vi "Shoot High Goal State Machine.vi"   [LabVIEW 2013]
uses:
  typedefs/fg_typedef.ctl
  typedefs/DevRef Type.ctl
  typedefs/subStates.ctl
  typedefs/singleUseSubstate.ctl
  <vilib>/Rock Robotics/WPI/Solenoid/WPI_SolenoidValue.ctl
  <vilib>/Rock Robotics/WPI/Solenoid/WPI_SolenoidGetEnum.vi
panel:
  # "A State Machine to Handle a High Goal Shot"
types:
  T1 = typedef "DevRef Type.ctl" = enum16{"Shooter Solenoid", "Latch Solenoid", "Right Up Sensor", "Right Down Sensor", "Hold Sensor", "2 Ball Switch", "Arm Encoder"}
  T2 = typedef "fg_typedef.ctl" = enum16{"Get", "Set"}
  T3 = typedef "subStates.ctl" = enum16{"null", "wait", "driver control", "auto", "manual override", "hold position", "rotate", "pickup", "pass", "load", "goto shoot", "shoot high goal", "shoot low goal", "cancel arm", "cancel shooter", "end"}
  T4 = typedef "WPI_SolenoidValue.ctl" = enum16{"Off", "On", "Forward", "Reverse"}
  T5 = typedef "singleUseSubstate.ctl" = enum16{"null", "wait", "shift high", "shift low", "extend shooter", "retract shooter", "latch", "unlatch", "end"}
  T6 = typedef "WPI_DigitalInputDevRef.ctl" = cluster{"DevStatus":errorcluster, "DIO Channel":T7, "Digital Module":T8}
  T7 = typedef "FPGA_DIOChannel.ctl" = enum8{"DIO 1", "DIO 2", "DIO 3", "DIO 4", "DIO 5", "DIO 6", "DIO 7", "DIO 8", "DIO 9", "DIO 10", "DIO 11", "DIO 12", "DIO 13", "DIO 14", "Invalid"}
  T8 = typedef "FPGA_TypedefDigitalModule.ctl" = enum16{"Digital Module 1", "Digital Module 2"}
  T9 = typedef "WPI_SolenoidDevRef.ctl" = cluster{"DevStatus":errorcluster, "Solenoid Module":T10, "Forward Solenoid Channel":T11, "Reverse Solenoid Channel":T11}
  T10 = typedef "FPGA_TypedefSolenoidModule.ctl" = enum16{"Solenoid Module 1", "Solenoid Module 2"}
  T11 = typedef "WPI_SolenoidChannel.ctl" = enum8{"Solenoid 1", "Solenoid 2", "Solenoid 3", "Solenoid 4", "Solenoid 5", "Solenoid 6", "Solenoid 7", "Solenoid 8", "Invalid"}
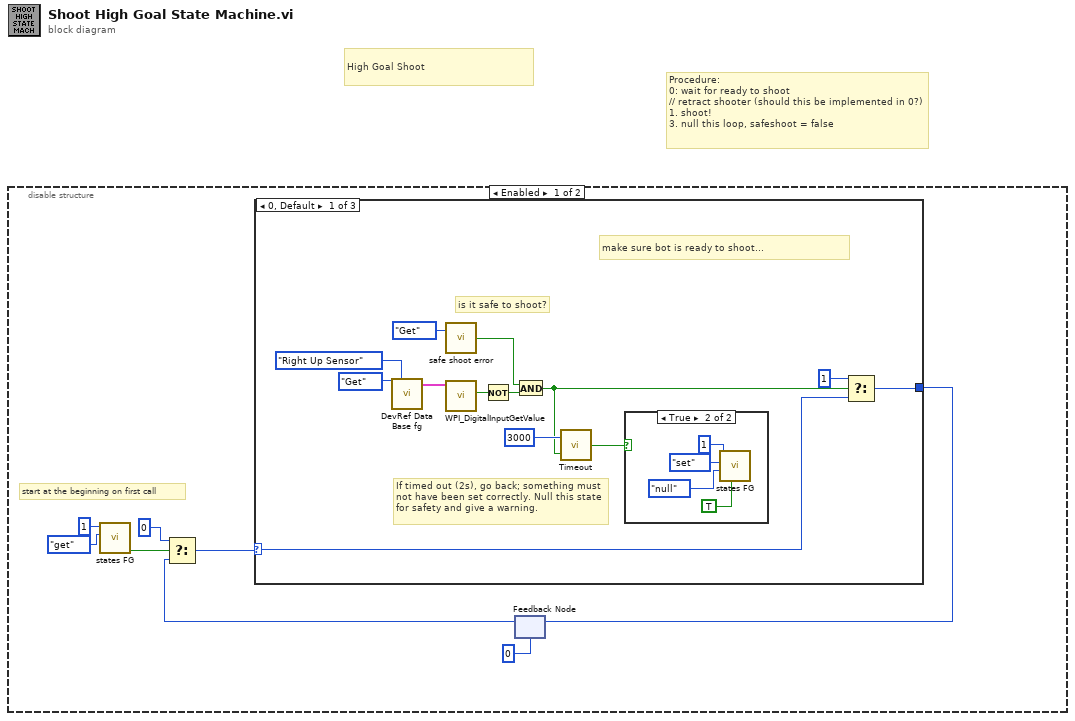
[diagram p0: block diagram]
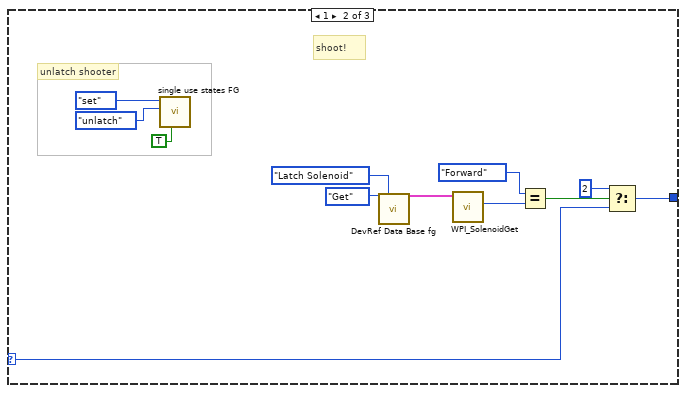
[diagram p3: hidden frame]
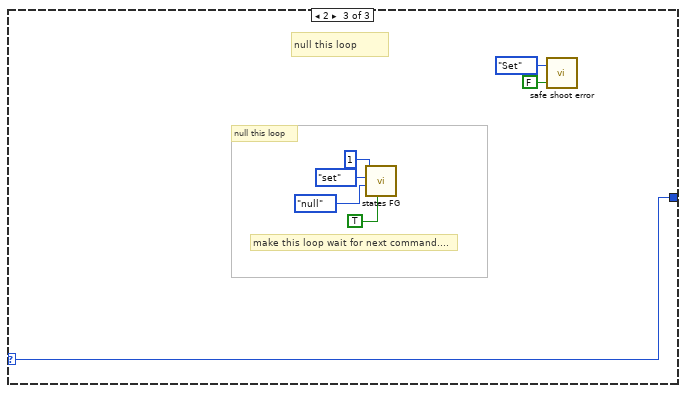
[diagram p4: hidden frame]
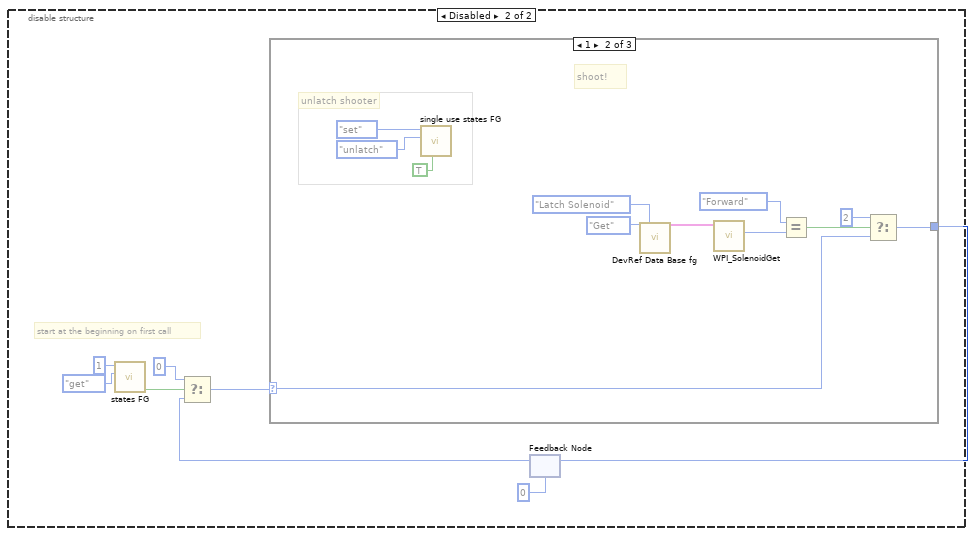
[diagram p5: hidden frame]
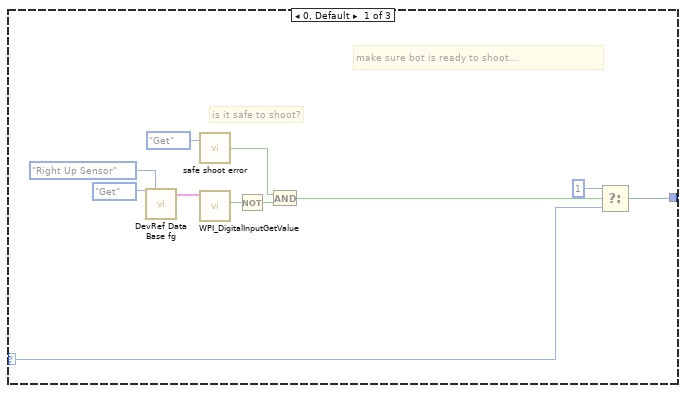
[diagram p6: hidden frame]
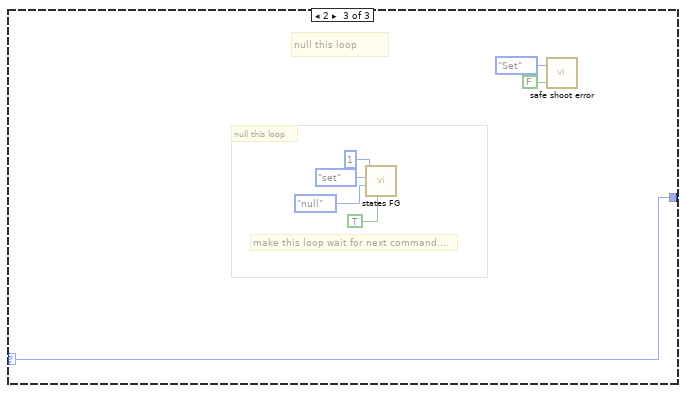
[diagram p7: hidden frame]
diagram:
  # "High Goal Shoot"
  # "Procedure:\n0: wait for ready to shoot\n// retract shooter (should this be implemented in 0?)\n1. shoot!\n3. null this loop, safeshoot = false"
  n1 = disable-structure shown="Enabled" {
    frame Enabled {
      # "start at the beginning on first call"
      n2 = call "states FG.vi"("menu (get)"=enum16{"set", "get"}."get", "Loop ID"=1) -> ("first call?"=w1:bool)  [unwired: 6 in, 3 out]
      n3 = feedback #1(u8 0) -> (w4:u8)
      n4 = Select(t=u8 0, s=w1, f=w4) -> (s? t:f=w3:u8)
      n5 = case shown="0, Default" w3 {
        selector: w3 -> [w19 w29 w44]
        tunnel: [w20 w28 w44] -> w7
        frame 0, Default {
          # "If timed out (2s), go back; something must\nnot have been set correctly. Null this state\nfor safety and give a warning."
          # "is it safe to shoot?"
          # "make sure bot is ready to shoot..."
          n6 = call "DevRef Data Base fg.vi"("Menu"=fg_typedef."Get", "DevRef to Get"=DevRef_Type."Right Up Sensor") -> ("Selected Sensor"=w17:T6)  [unwired: 23 in, 2 out]
          n7 = call "safe shoot error.vi"("Menu"=fg_typedef."Get") -> ("Can Shoot Safely?"=w15:bool)  [unwired: 1 in]
          n8 = call <vilib>:"WPI_DigitalInputGetValue.vi"("DigitalInputDevRef"=w17) -> ("Value"=w21:bool)  [unwired: 8 in, 2 out]
          n9 = Not(x=w21) -> (.not. x?=w14:bool)
          n10 = And(x=w15, y=w14) -> (x .and. y?=w9:bool)
          n11 = call "Timeout.vi"("Done with Task?"=w9, "Timeout (ms)"=u32 3000) -> ("Timed Out?"=w10:bool)  [unwired: 1 in]
          n12 = case shown="True" w10 {
            frame False {
            }
            frame True {
              n13 = call "states FG.vi"("exit in"=TRUE, "subState in"=subStates."null", "menu (get)"=enum16{"set", "get"}."set", "Loop ID"=1) -> ()  [unwired: 4 in, 4 out]
            }
          }
          n14 = Select(t=u8 1, s=w9, f=w19) -> (s? t:f=w20:u8)
        }
        frame 1 {
          # "unlatch shooter"
          # "shoot!"
          n15 = call "single use states FG.vi"("exit in"=TRUE, "substate"=singleUseSubstate."unlatch", "menu (get)"=enum16{"set", "get"}."set") -> ()  [unwired: 5 in, 4 out]
          n16 = call "DevRef Data Base fg.vi"("Menu"=fg_typedef."Get", "DevRef to Get"=DevRef_Type."Latch Solenoid") -> ("Selected Solenoid"=w33:T9)  [unwired: 23 in, 2 out]
          n17 = call-poly <vilib>:"WPI_SolenoidGet.vi"("SolenoidDevRef"=w33) -> ("Value"=w32:T4)  [unwired: 8 in, 2 out]
          n18 = Equal?(x=WPI_SolenoidValue."Forward" ("Value"), y=w32) -> (x = y?=w30:bool)
          n19 = Select(t=u8 2, s=w30, f=w29) -> (s? t:f=w28:u8)
        }
        frame 2 {
          # "null this loop"
          # "null this loop"
          # "make this loop wait for next command...."
          n20 = call "states FG.vi"("exit in"=TRUE, "subState in"=subStates."null", "menu (get)"=enum16{"set", "get"}."set", "Loop ID"=1) -> ()  [unwired: 4 in, 4 out]
          n21 = call "safe shoot error.vi"("Can Shoot Safely?"=FALSE, "Menu"=fg_typedef."Set") -> ()  [unwired: 1 out]
        }
      }
      n22 = feedback-in #1(w7) -> ()
    }
    frame Disabled {
      # "start at the beginning on first call"
      n23 = call "states FG.vi"("menu (get)"=enum16{"set", "get"}."get", "Loop ID"=1) -> ("first call?"=w45:bool)  [unwired: 6 in, 3 out]
      n24 = feedback #2(u8 0) -> (w48:u8)
      n25 = Select(t=u8 0, s=w45, f=w48) -> (s? t:f=w47:u8)
      n26 = case shown="1" w47 {
        selector: w47 -> [w61 w67 w82]
        tunnel: [w62 w66 w82] -> w51
        frame 0, Default {
          # "is it safe to shoot?"
          # "make sure bot is ready to shoot..."
          n27 = call "DevRef Data Base fg.vi"("Menu"=fg_typedef."Get", "DevRef to Get"=DevRef_Type."Right Up Sensor") -> ("Selected Sensor"=w59:T6)  [unwired: 23 in, 2 out]
          n28 = call "safe shoot error.vi"("Menu"=fg_typedef."Get") -> ("Can Shoot Safely?"=w57:bool)  [unwired: 1 in]
          n29 = call <vilib>:"WPI_DigitalInputGetValue.vi"("DigitalInputDevRef"=w59) -> ("Value"=w63:bool)  [unwired: 8 in, 2 out]
          n30 = Not(x=w63) -> (.not. x?=w56:bool)
          n31 = And(x=w57, y=w56) -> (x .and. y?=w53:bool)
          n32 = Select(t=u8 1, s=w53, f=w61) -> (s? t:f=w62:u8)
        }
        frame 1 {
          # "unlatch shooter"
          # "shoot!"
          n33 = call "single use states FG.vi"("exit in"=TRUE, "substate"=singleUseSubstate."unlatch", "menu (get)"=enum16{"set", "get"}."set") -> ()  [unwired: 5 in, 4 out]
          n34 = call "DevRef Data Base fg.vi"("Menu"=fg_typedef."Get", "DevRef to Get"=DevRef_Type."Latch Solenoid") -> ("Selected Solenoid"=w71:T9)  [unwired: 23 in, 2 out]
          n35 = call-poly <vilib>:"WPI_SolenoidGet.vi"("SolenoidDevRef"=w71) -> ("Value"=w70:T4)  [unwired: 8 in, 2 out]
          n36 = Equal?(x=WPI_SolenoidValue."Forward" ("Value"), y=w70) -> (x = y?=w68:bool)
          n37 = Select(t=u8 2, s=w68, f=w67) -> (s? t:f=w66:u8)
        }
        frame 2 {
          # "null this loop"
          # "null this loop"
          # "make this loop wait for next command...."
          n38 = call "states FG.vi"("exit in"=TRUE, "subState in"=subStates."null", "menu (get)"=enum16{"set", "get"}."set", "Loop ID"=1) -> ()  [unwired: 4 in, 4 out]
          n39 = call "safe shoot error.vi"("Can Shoot Safely?"=FALSE, "Menu"=fg_typedef."Set") -> ()  [unwired: 1 out]
        }
      }
      n40 = feedback-in #2(w51) -> ()
    }
  }
